vi "parse extended err JSON.vi"(8 "error in (no error)":errorcluster, 11 "JSON string in":string) -> (0 "error out":errorcluster, 3 "stack trace":T1[](array[typedef]))   [LabVIEW 2018, in "LV-Julia_ZMQ-Roundtrip_lib.lvlib"]
uses:
  LV-Julia_ZMQ-Roundtrip_lib.lvlib
  StackFrame.ctl
  extended error cluster.ctl
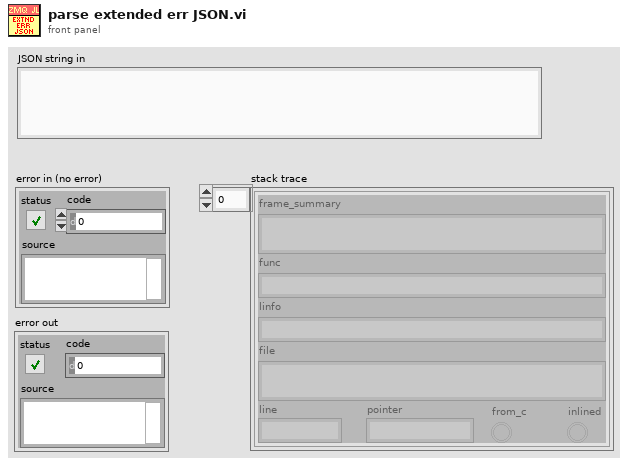
[diagram p1: front panel]
types:
  T1 = typedef "LV-Julia_ZMQ-Roundtrip_lib.lvlib/StackFrame.ctl" = cluster{"frame_summary":string, "func":string, "linfo":string, "file":string, "line":i32, "pointer":u64, "from_c":bool, "inlined":bool}
  T2 = typedef "LV-Julia_ZMQ-Roundtrip_lib.lvlib/extended error cluster.ctl" = cluster{"errorinfo":cluster{"status":bool, "code":i32, "source":string, "stack_trace":T1[]}}
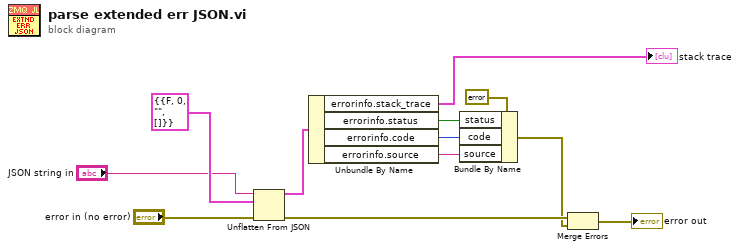
[diagram p0: block diagram]
diagram:
  n1 = Unflatten From JSON(JSON string="JSON string in", type and defaults=T2 {"errorinfo"={"status"=FALSE, "code"=0, "source"="", "stack_trace"=[]}} ("extended error"), error in (no error)="error in (no error)") -> (value=w12:T2, error out=w10:errorcluster)  [unwired: 4 in]
  n2 = Unbundle By Name(w12) -> ("errorinfo.stack_trace"=→"stack trace":T1[], "errorinfo.status"=w4:bool, "errorinfo.code"=w5:i32, "errorinfo.source"=w6:string)
  n3 = Bundle By Name(cluster=errorcluster {"status"=FALSE, "code"=0, "source"=""} ("input cluster"), "status"=w4, "code"=w5, "source"=w6) -> (w2:errorcluster)
  n4 = Merge Errors(w10, w2) -> (→"error out":errorcluster)
